vi "Ic_LaguerreGaussMode.vi"(6 "Pixel Pitch 0:20um_or_ 1:12.5um":u8, 7 "Beam size / mm":dbl=1.0, 8 "error in (no error)":errorcluster, 9 "m :azimuthal index":u32, 10 "p :radial index":u32, 11 "2D array in (LCOS size buf)":u8[][](array[numeric])) -> (0 "error out":errorcluster, 3 "2D array out":u8[][](array[numeric]))   [LabVIEW 2015]
uses:
  SLM_Control_VI_source/Image_Control.dll
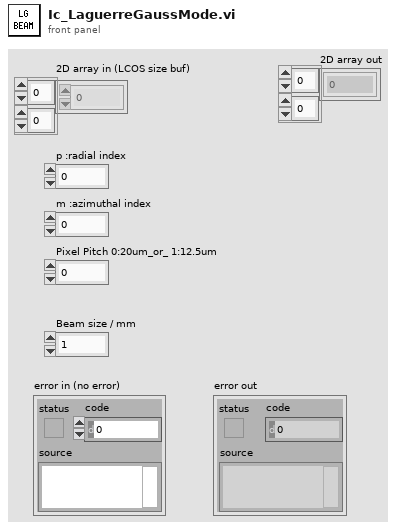
[diagram p1: front panel]
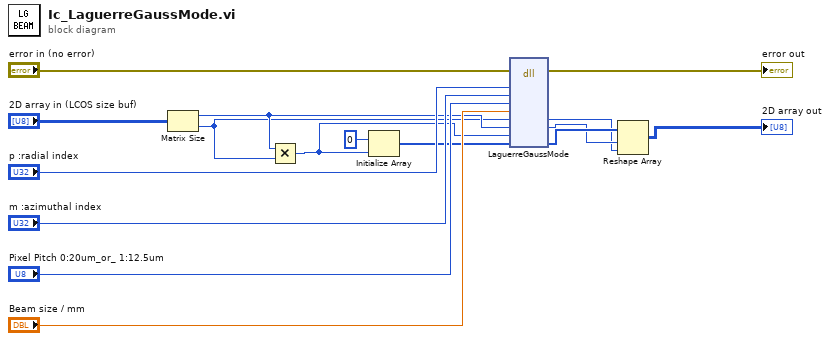
[diagram p0: block diagram]
diagram:
  n1 = Matrix Size(0:"2D array in (LCOS size buf)") -> (1:w8:i32, 2:w7:i32)
  n2 = Multiply(x=w8, y=w7) -> (x*y=w5:i32)
  n3 = Initialize Array(u8 0 ("要素"), w5) -> (w6:u8[])
  n4 = dll-call lib="C:/Users/hs5921/Desktop/SLM_Control_VI_source/Image_Control.dll" fn="LaguerreGaussMode"(error in="error in (no error)", "p"="p :radial index", "m"="m :azimuthal index", "PixelPitch0:20um_or_1:12.5um"="Pixel Pitch 0:20um_or_ 1:12.5um", "BeamSizeMm"="Beam size / mm", "X_pixel_target"=w7, "Y_pixel_target"=w8, "targetDataSize"=w5, "1DArrayOut"=w6) -> (error out=→"error out":errorcluster, "X_pixel_target"=w2:i32, "Y_pixel_target"=w3:i32, "1DArrayOut"=w4:u8[])  [unwired: 8 in, 1 out]
  n5 = Reshape Array(w4, w3, w2) -> (→"2D array out":u8[][])
